vi "CVT1NamedReadTest.vi"() -> (3 "Unit Test Framework Results":T1)   [LabVIEW 2013, in "UnitTests.lvlib"]
uses:
  UnitTests.lvlib
  <vilib>/utf/common/utf_test_result_troll.ctl
  <vilib>/utf/common/utf_test_result.ctl
  <vilib>/utf/common/utf_test_result_failure.ctl
  <vilib>/utf/common/utf_test_comparison_operators.ctl
  <vilib>/utf/common/utf_vi_tag.ctl
  <vilib>/NI/Current Value Table/Read.vi
  <vilib>/NI/Current Value Table/DataTypes/I32_Read.vi
  <vilib>/NI/Current Value Table/Type to Enum.vi
  <vilib>/NI/Current Value Table/DataTypes/I32_Type To Enum.vi
  <vilib>/NI/Current Value Table/Compatibility/TagConverter.vi
  <vilib>/NI/Current Value Table/Create Tags.vi
  <vilib>/NI/Current Value Table/FGVs/CVT Globals.vi
  <vilib>/NI/Current Value Table/FGVs/Tag Memory.vi
  <vilib>/NI/Current Value Table/Memory Block.vi
  <vilib>/NI/Current Value Table/DataTypes/I32_Memory Block.vi
  <vilib>/utf/NI_UnitTestFramework.lvlib
panel:
  out "Value":i32
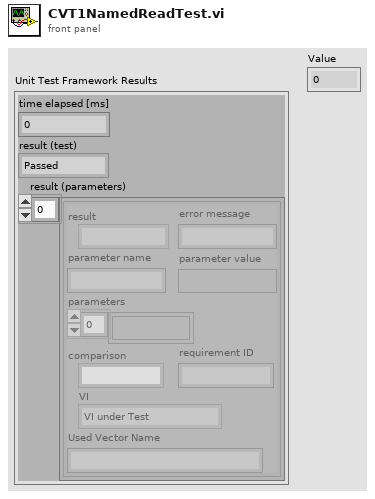
[diagram p1: front panel]
types:
  T1 = typedef "NI_UnitTestFramework.lvlib/utf_test_result_troll.ctl" = cluster{"time elapsed [ms]":u32, "result (test)":T2, "result (parameters)":T3[]}
  T2 = typedef "NI_UnitTestFramework.lvlib/utf_test_result.ctl" = enum16{"Passed", "Failed", "Error", "Skipped", "Not Processed"}
  T3 = typedef "NI_UnitTestFramework.lvlib/utf_test_result_failure.ctl" = cluster{"result":T2, "error message":string, "parameter name":string, "parameter value":variant, "parameters":variant[], "comparison":T4, "requirement ID":string, "VI":T5, "Used Vector Name":string}
  T4 = typedef "NI_UnitTestFramework.lvlib/utf_test_comparison_operators.ctl" = enum16{"=", "!=", ">", ">=", "<", "<=", "range", "symmetric tolerance", "asymmetric tolerance", "string contains", "string not contain", "array size", "string length", "array range", "by element", "array range (limit array)", "user-defined", "array contains", "array not contain", "vector length", "= (elm)", "!= (elm)", "= (case insensitive)", "!= (case insensitive)"}
  T5 = typedef "NI_UnitTestFramework.lvlib/utf_vi_tag.ctl" = enum16{"Setup VI", "VI under Test", "Teardown VI"}
  T6 = typedef "cvt_Tag Configuration.ctl" = cluster{"Name":string, "Data Type":T7, "Array":bool, "Size":u32, "Default":string, "Enum":string[], "Description":string}
  T7 = typedef "cvt_Data Types.ctl" = enum16{"Bool", "U8", "I32", "Double", "String", "Enum"}
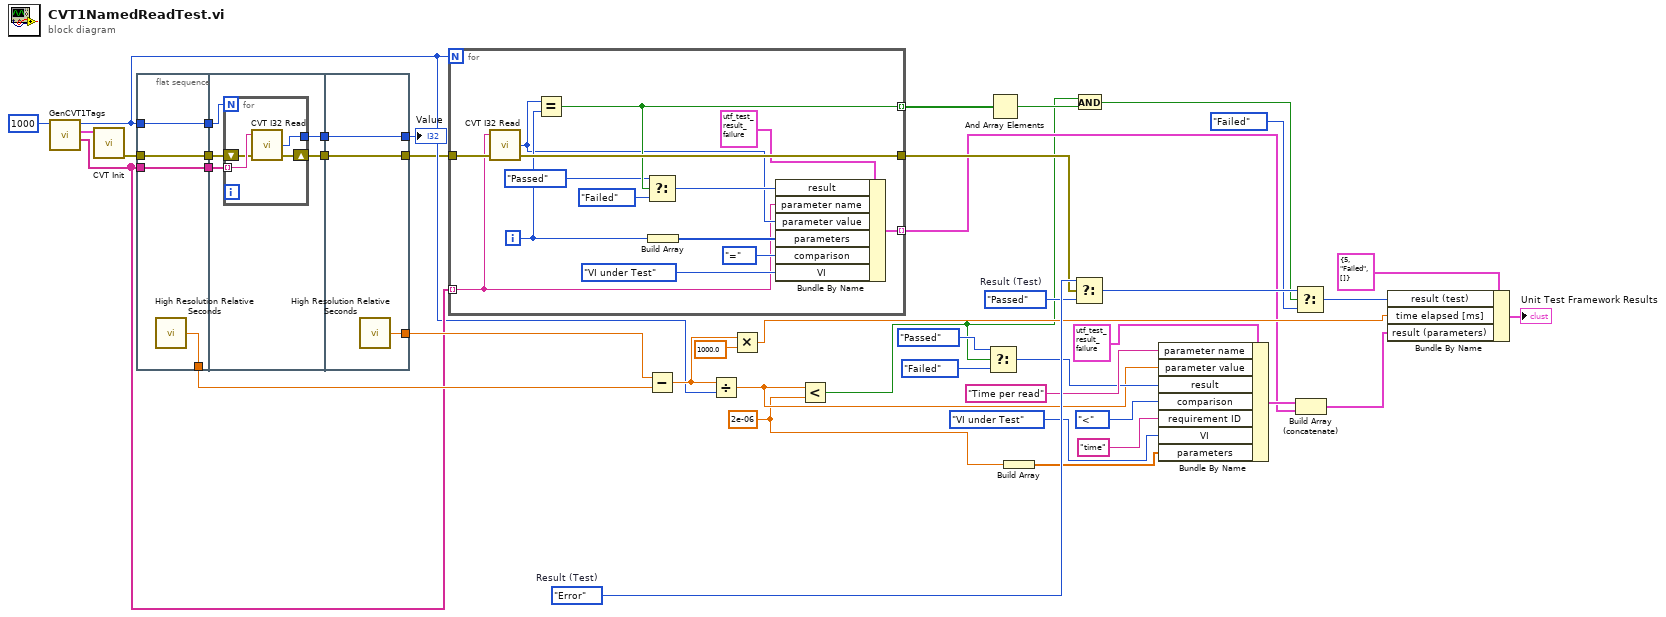
[diagram p0: block diagram]
diagram:
  w7 = 2e-06 ("y")
  w38 = utf_test_result."Error"  # Result (Test)
  w37 = utf_test_result."Passed"  # Result (Test)
  n1 = call "GenCVT1Tags.vi"("Number of Tags in"=1000) -> ("Names"=w23:string[], "Tags"=w31:T6[], "Number of Tags out"=w22:i32)  [unwired: 8 in]
  n2 = call <vilib>:"CVT Init.vi"("Tag List"=w31) -> ("error out"=w30:errorcluster)  [unwired: 10 in]
  n3 = flat-sequence {
    tunnel: [w47] -> w40
    tunnel: w30 -> [w44]
    tunnel: [w46] -> w29
    tunnel: w22 -> [w46]
    tunnel: w23 -> [w45]
    tunnel: [w45] -> w28
    tunnel: [w44] -> w27
    tunnel: w29 -> [w52]
    tunnel: w28 -> [w51]
    tunnel: w27 -> [w50]
    tunnel: [w49] -> w26
    tunnel: [w48] -> w2
    tunnel: [w59] -> w41
    tunnel: w26 -> [w58]
    tunnel: [w58] -> w21
    tunnel: [w57] -> w1
    tunnel: w2 -> [w57]
    frame #0 {
      n4 = call <vilib>:"High Resolution Relative Seconds.vi"() -> ("relative seconds"=w47:dbl)
    }
    frame #1 {
      n5 = for {
        N: w52 -> [_]
        tunnel: w51 -> [w56] mode=indexing
        shift-right: [w54] -> w49
        shift-left: w50 -> [w55]
        tunnel: [w53] -> w48
        n6 = call <vilib>:"CVT I32 Read.vi"("error in (no error)"=w55, "Tag Name"=w56) -> ("error out"=w54:errorcluster, "Value"=w53:i32)  [unwired: 2 in]
      }
    }
    frame #2 {
      n7 = call <vilib>:"High Resolution Relative Seconds.vi"() -> ("relative seconds"=w59:dbl)
    }
  }
  n8 = for {
    N: w22 -> [_]
    tunnel: w23 -> [w60] mode=indexing
    tunnel: w21 -> [w73]
    tunnel: [w72] -> w20
    tunnel: [w69] -> w19 mode=indexing
    tunnel: [w65] -> w5 mode=indexing
    i -> [w62]
    n9 = call <vilib>:"CVT I32 Read.vi"("error in (no error)"=w73, "Tag Name"=w60) -> ("error out"=w72:errorcluster, "Value"=w61:i32)  [unwired: 2 in]
    n10 = Equal?(x=w61, y=w62) -> (x = y?=w69:bool)
    n11 = Select(t=utf_test_result."Passed" ("result"), s=w69, f=utf_test_result."Failed" ("result")) -> (s? t:f=w66:T2)
    n12 = Build Array(w62) -> (w63:i32[])
    n13 = Bundle By Name(cluster=T3 {"result"=enum."Passed", "error message"="", "parameter name"="", "parameter value"=variant, "parameters"=[], "comparison"=enum."=", "requirement ID"="", "VI"=enum."Setup VI", "Used Vector Name"=""} ("Unit Test Framework - result (parameters)"), "result"=w66, "parameter name"=w60, "parameter value"=w61, "parameters"=w63, "comparison"=utf_test_comparison_operators."=", "VI"=utf_vi_tag."VI under Test") -> (w65:T3)
  }
  n14 = Subtract(x=w41, y=w40) -> (x-y=w25:dbl)
  n15 = Divide(x=w25, y=w22) -> (x/y=w10:dbl)
  n16 = Multiply(x=w25, y=1000.0) -> (x*y=w32:dbl)
  n17 = Less?(x=w10, y=w7) -> (x < y?=w3:bool)
  n18 = Select(t=utf_test_result."Passed" ("result"), s=w3, f=utf_test_result."Failed" ("result")) -> (s? t:f=w11:T2)
  n19 = And Array Elements(Boolean array=w19) -> (logical AND=w18:bool)
  n20 = Build Array(w7) -> (w6:dbl[])
  n21 = Select(t=w38, s=w20, f=w37) -> (s? t:f=w17:T2)
  n22 = And(x=w3, y=w18) -> (x .and. y?=w4:bool)
  n23 = Bundle By Name(cluster=T3 {"result"=enum."Passed", "error message"="", "parameter name"="", "parameter value"=variant, "parameters"=[], "comparison"=enum."=", "requirement ID"="", "VI"=enum."Setup VI", "Used Vector Name"=""} ("Unit Test Framework - result (parameters)"), "parameter name"="Time per read", "parameter value"=w10, "result"=w11, "comparison"=utf_test_comparison_operators."<", "requirement ID"="time", "VI"=utf_vi_tag."VI under Test", "parameters"=w6) -> (w35:T3)
  n24 = Select(t=w17, s=w4, f=utf_test_result."Failed") -> (s? t:f=w15:T2)
  n25 = Build Array (concatenate)(w35, w5) -> (w34:T3[])
  n26 = Bundle By Name(cluster=T1 {"time elapsed [ms]"=5, "result (test)"=enum."Failed", "result (parameters)"=[]} ("Unit Test Framework - Result"), "result (test)"=w15, "time elapsed [ms]"=w32, "result (parameters)"=w34) -> (→"Unit Test Framework Results":T1)
  "Value" <- w1
